vi "Data Analysis.Convert JSON to 2D.vi"(11 "Test Result V2":T1={"Type"="Test Data", "Version"="1.0.0", "TestEvent"={"ProcessStep"="", "StartTime"="", "EndTime"="", "Mode"="", "Operator"="", "Comment"="", "Result"={"State"="", "Code"=0, "Desc"="", "Details"=""}}, "UUTInfo"={"Product"="", "Description"="", "PN"="", "SN"="", "LotNumber"="", "DateCode"="", "AltID"="", "Revision"="", "Properties"=[]}, "Station"={"Name"="", "Location"="", "ConfigID"="", "PCName"="", "Slot"=""}, "TestSequence"={"Name"="", "Setup"=[]}, "ResultData"=[], "DataObjs"=[]}) -> (3 "2D":string[][](array[string]))   [LabVIEW 2018]
uses:
  Common/Utils/Reports/Report.Result Data JSON V2.0.0.ctl
  Common/Utils/Reports/Report.Result Test Event.ctl
  Common/Utils/Reports/Report.Result State.ctl
  Common/Utils/Reports/Report.Result UUTInfo.ctl
  Common/Utils/Reports/Report.Result Test Station.ctl
  Common/Utils/Reports/Report.Result Test Sequence.ctl
  Common/Utils/Reports/Report.Result Measurement JSON Safe.ctl
  Common/Utils/Reports/Report.Result DataObject.ctl
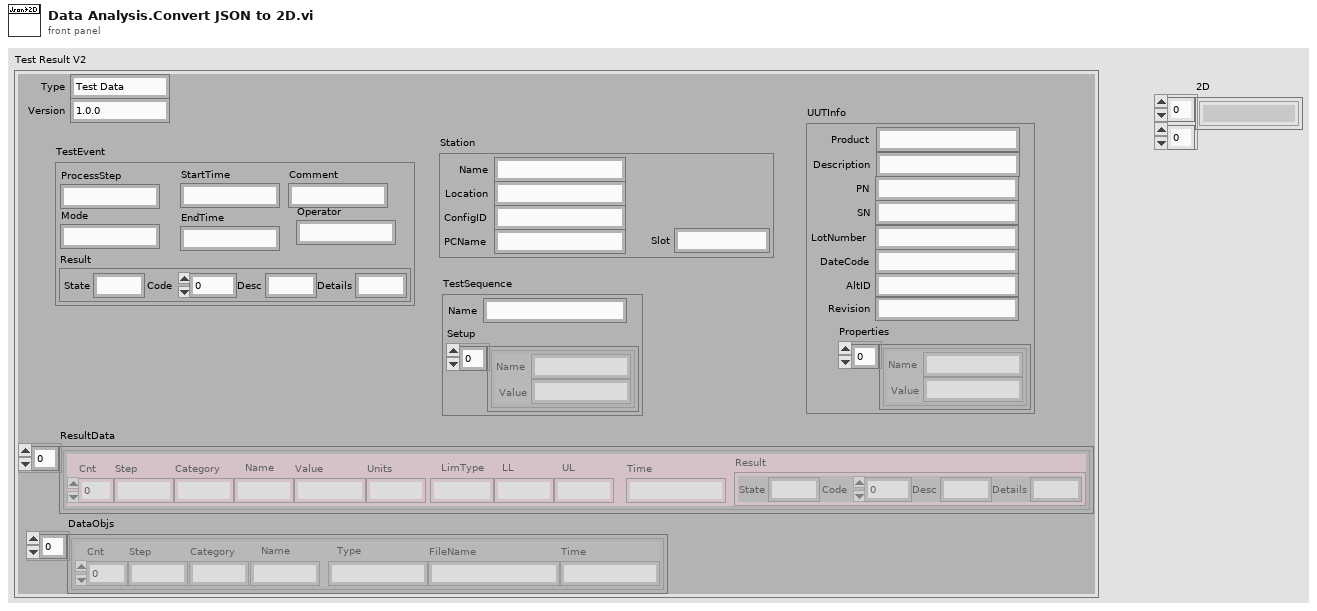
[diagram p1: front panel]
types:
  T1 = typedef "Report.Result Data JSON V2.0.0.ctl" = cluster{"Type":string, "Version":string, "TestEvent":T2, "UUTInfo":T4, "Station":T5, "TestSequence":T6, "ResultData":T7[], "DataObjs":T8[]}
  T2 = typedef "Report.Result Test Event.ctl" = cluster{"ProcessStep":string, "StartTime":string, "EndTime":string, "Mode":string, "Operator":string, "Comment":string, "Result":T3}
  T3 = typedef "Report.Result State.ctl" = cluster{"State":string, "Code":i32, "Desc":string, "Details":string}
  T4 = typedef "Report.Result UUTInfo.ctl" = cluster{"Product":string, "Description":string, "PN":string, "SN":string, "LotNumber":string, "DateCode":string, "AltID":string, "Revision":string, "Properties":cluster{"Name":string, "Value":string}[]}
  T5 = typedef "Report.Result Test Station.ctl" = cluster{"Name":string, "Location":string, "ConfigID":string, "PCName":string, "Slot":string}
  T6 = typedef "Report.Result Test Sequence.ctl" = cluster{"Name":string, "Setup":cluster{"Name":string, "Value":string}[]}
  T7 = typedef "Report.Result Measurement JSON Safe.ctl" = cluster{"Cnt":i32, "Step":string, "Category":string, "Name":string, "Value":string, "Units":string, "LimType":string, "LL":string, "UL":string, "Time":string, "Result":T3}
  T8 = typedef "Report.Result DataObject.ctl" = cluster{"Cnt":i32, "Step":string, "Category":string, "Name":string, "Type":string, "FileName":string, "Time":string}
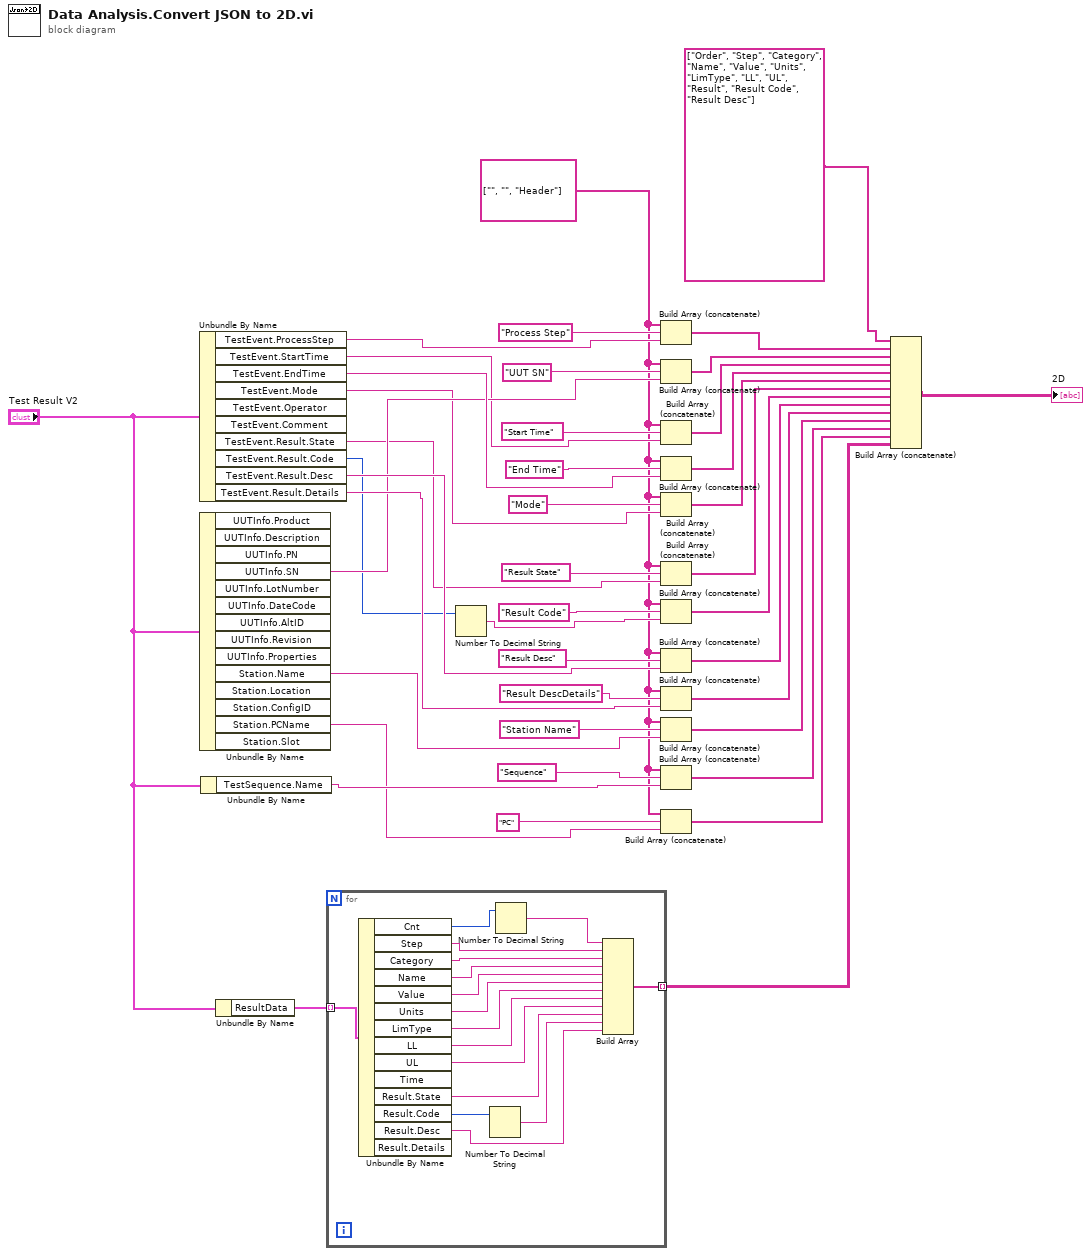
[diagram p0: block diagram]
diagram:
  w3 = string[] ["", "", "Header"]
  n1 = Unbundle By Name("Test Result V2") -> ("TestEvent.ProcessStep"=w23:string, "TestEvent.StartTime"=w22:string, "TestEvent.EndTime"=w25:string, "TestEvent.Mode"=w21:string, "TestEvent.Result.State"=w20:string, "TestEvent.Result.Code"=w19:i32, "TestEvent.Result.Desc"=w33:string, "TestEvent.Result.Details"=w32:string)  [unwired: 2 out]
  n2 = Unbundle By Name("Test Result V2") -> ("UUTInfo.SN"=w24:string, "Station.Name"=w36:string, "Station.PCName"=w35:string)  [unwired: 11 out]
  n3 = Unbundle By Name("Test Result V2") -> ("TestSequence.Name"=w38:string)
  n4 = Unbundle By Name("Test Result V2") -> ("ResultData"=w4:T7[])
  n5 = for {
    tunnel: w4 -> [w59] mode=indexing
    tunnel: [w44] -> w1 mode=indexing
    n6 = Unbundle By Name(w59) -> ("Cnt"=w58:i32, "Step"=w56:string, "Category"=w55:string, "Name"=w54:string, "Value"=w53:string, "Units"=w52:string, "LimType"=w51:string, "LL"=w50:string, "UL"=w49:string, "Result.State"=w47:string, "Result.Code"=w48:i32, "Result.Desc"=w45:string)  [unwired: 2 out]
    n7 = Number To Decimal String(number=w48) -> (decimal integer string=w46:string)  [unwired: 1 in]
    n8 = Number To Decimal String(number=w58) -> (decimal integer string=w57:string)  [unwired: 1 in]
    n9 = Build Array(w57, w56, w55, w54, w53, w52, w51, w50, w49, w47, w46, w45) -> (w44:string[])
  }
  n10 = Number To Decimal String(number=w19) -> (decimal integer string=w18:string)  [unwired: 1 in]
  n11 = Build Array (concatenate)(w3, "Process Step", w23) -> (w17:string[])
  n12 = Build Array (concatenate)(w3, "UUT SN", w24) -> (w16:string[])
  n13 = Build Array (concatenate)(w3, "Start Time", w22) -> (w15:string[])
  n14 = Build Array (concatenate)(w3, "End Time", w25) -> (w14:string[])
  n15 = Build Array (concatenate)(w3, "Mode", w21) -> (w13:string[])
  n16 = Build Array (concatenate)(w3, "Result State", w20) -> (w12:string[])
  n17 = Build Array (concatenate)(w3, "Result Code", w18) -> (w11:string[])
  n18 = Build Array (concatenate)(w3, "Result Desc", w33) -> (w10:string[])
  n19 = Build Array (concatenate)(w3, "Result DescDetails", w32) -> (w9:string[])
  n20 = Build Array (concatenate)(w3, "Station Name", w36) -> (w8:string[])
  n21 = Build Array (concatenate)(w3, "Sequence", w38) -> (w7:string[])
  n22 = Build Array (concatenate)(w3, "PC", w35) -> (w6:string[])
  n23 = Build Array (concatenate)(string[] ["Order", "Step", "Category", "Name", "Value", "Units", "LimType", "LL", "UL", "Result", "Result Code", "Result Desc"], w17, w16, w15, w14, w13, w12, w11, w10, w9, w8, w7, w6, w1) -> (→"2D":string[][])
